vi "CIMAQ_StdDev.vi"(6 "Window Size":i32=3, 7 "Variance(F) /StdDev":bool, 8 "error in":errorcluster, 9 "Dst(optional)":T1, 11 "Src":T1) -> (0 "error out":errorcluster, 3 "Result":T1)   [LabVIEW 2017]
doc: "Computes the local variance of the image as the difference between the mean of the local squares and the square of the local means."
uses:
  <vilib>/vision/Image Controls.llb/IMAQ Image.ctl
  <vilib>/vision/NI_Vision_Development_Module.lvlib
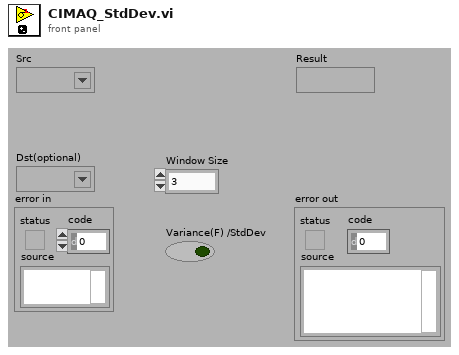
[diagram p1: front panel]
types:
  T1 = typedef "IMAQ Image.ctl" = refnum<image>
  T2 = typedef "Image Type" = u32
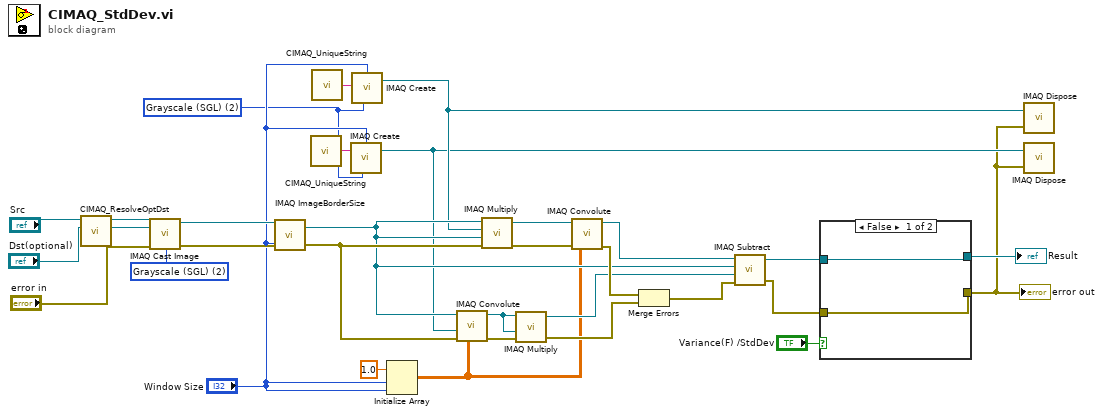
[diagram p0: block diagram]
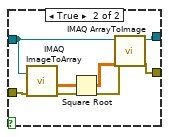
[diagram p2: hidden frame]
diagram:
  w8 = T2 2 items=["Grayscale (U8)", "Grayscale (I16)", "Grayscale (SGL)", "Complex (CSG)", "RGB (U32)", "HSL (U32)", "RGB (U64)", "Grayscale (U16)"] ("Image Type")
  w14 = T2 2 items=["Grayscale (U8)", "Grayscale (I16)", "Grayscale (SGL)", "Complex (CSG)", "RGB (U32)", "HSL (U32)", "RGB (U64)", "Grayscale (U16)"] ("Image Type")
  n1 = call "CIMAQ_ResolveOptDst.vi"("Dst(optional)"="Dst(optional)", "Src"="Src") -> ("Dst"=w9:T1, "Src"=w10:T1)  [unwired: 7 in]
  n2 = call "IMAQ Cast Image"("Image Type"=w14, "error in (no error)"="error in", "Image Dst"=w9, "Image Src"=w10) -> ("error out"=w19:errorcluster, "Image Dst Out"=w21:T1)  [unwired: 2 in, 4 out]
  n3 = call "IMAQ ImageBorderSize"("Image"=w21, "Image border size in"="Window Size", "error in (no error)"=w19) -> ("Image Out"=w20:T1, "error out"=w32:errorcluster)  [unwired: 1 in, 1 out]
  n4 = call <userlib>:"CIMAQ_UniqueString.vi"() -> ("String"=w15:string)  [unwired: 5 in]
  n5 = call <userlib>:"CIMAQ_UniqueString.vi"() -> ("String"=w16:string)  [unwired: 5 in]
  n6 = call "IMAQ Create"("Border Size"="Window Size", "Image Name"=w15, "Image Type"=w8) -> ("New Image"=w6:T1)  [unwired: 2 in, 1 out]
  n7 = call "IMAQ Create"("Border Size"="Window Size", "Image Name"=w16, "Image Type"=w8) -> ("New Image"=w7:T1)  [unwired: 2 in, 1 out]
  n8 = Initialize Array(sgl 1.0 ("element"), "Window Size", "Window Size") -> (w17:sgl[][])
  n9 = call "IMAQ Convolute"("Kernel"=w17, "error in (no error)"=w32, "Image Dst"=w6, "Image Src"=w20) -> ("error out"=w27:errorcluster, "Image Dst Out"=w26:T1)  [unwired: 3 in, 3 out]
  n10 = call "IMAQ Multiply"("Image Src A"=w20, "Image Dst"=w7, "Image Src B"=w20, "error in (no error)"=w32) -> ("Image Dst Out"=w25:T1, "error out"=w28:errorcluster)  [unwired: 1 in, 2 out]
  n11 = call "IMAQ Multiply"("Image Src A"=w26, "Image Src B"=w26, "error in (no error)"=w27) -> ("Image Dst Out"=w30:T1, "error out"=w24:errorcluster)  [unwired: 2 in, 2 out]
  n12 = call "IMAQ Convolute"("Kernel"=w17, "error in (no error)"=w28, "Image Src"=w25) -> ("error out"=w31:errorcluster, "Image Dst Out"=w29:T1)  [unwired: 4 in, 3 out]
  n13 = Merge Errors(w31, w24) -> (w23:errorcluster)
  n14 = call "IMAQ Subtract"("Image Src A"=w29, "Image Dst"=w20, "Image Src B"=w30, "error in (no error)"=w23) -> ("Image Dst Out"=w5:T1, "error out"=w3:errorcluster)  [unwired: 1 in, 2 out]
  n15 = case shown="False" "Variance(F) /StdDev" {
    tunnel: w5 -> [w34 w35]
    tunnel: [w34 w39] -> w4
    tunnel: w3 -> [w33 w38]
    tunnel: [w33 w36] -> w2
    frame False {
    }
    frame True {
      n16 = call "IMAQ ImageToArray"("error in (no error)"=w38, "Image"=w35) -> ("Image Pixels (Float)"=w40:sgl[][], "error out"=w37:errorcluster)  [unwired: 2 in, 3 out]
      n17 = Square Root(x=w40) -> (sqrt(x)=w41:sgl[][])
      n18 = call "IMAQ ArrayToImage"("Image Pixels (Float)"=w41, "error in (no error)"=w37, "Image"=w35) -> ("error out"=w36:errorcluster, "Image Out"=w39:T1)  [unwired: 7 in]
    }
  }
  "error out" <- w2
  "Result" <- w4
  n19 = call "IMAQ Dispose"("Image"=w7, "error in (no error)"=w2) -> ()  [unwired: 4 in, 1 out]
  n20 = call "IMAQ Dispose"("Image"=w6, "error in (no error)"=w2) -> ()  [unwired: 4 in, 1 out]
